vi "Basic Sweep.vi"(8 "error in (no error)":errorcluster, 11 "Wavepond in":refnum<class "Wavepond.lvclass">) -> (0 "error out":errorcluster, 3 "Wavepond out":refnum<class "Wavepond.lvclass">)   [LabVIEW 2015, in "Wavepond.lvclass"]
uses:
  Wavepond.lvclass
  Wavepond Commands.ctl
  Wavepond.lvclass/Wavepond.ctl
panel:
  out "standard output":string
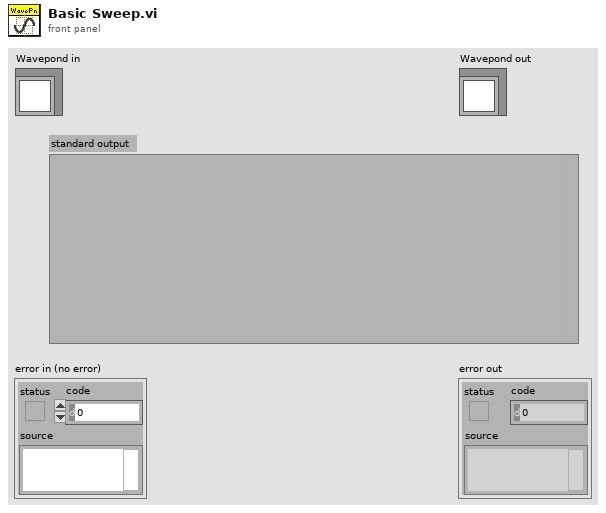
[diagram p1: front panel]
types:
  T1 = typedef "Wavepond.lvclass/Wavepond Commands.ctl" = enum16{"Initialize", "SetFrequency", "SetAtten", "WriteData", "EnableSweep", "SetLoopCnt", "SetClkDiv", "SelExtTrig", "SoftTrig", "En_SqWave"}
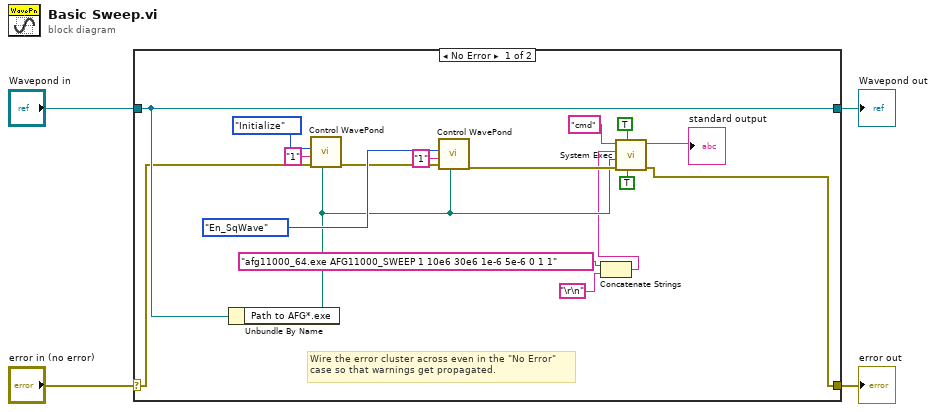
[diagram p0: block diagram]
diagram:
  n1 = case shown="No Error" "error in (no error)" {
    selector: "error in (no error)" -> [w19 w23]
    tunnel: [w10 w23] -> w3
    tunnel: [w21 w22] -> w1
    tunnel: "Wavepond in" -> [w21 w22]
    frame No Error {
      # "Wire the error cluster across even in the \"No Error\"\ncase so that warnings get propagated."
      n2 = Unbundle By Name(w21) -> ("Path to AFG*.exe"=w11:path)
      n3 = call "Control WavePond.vi"("working directory"=w11, "Error In"=w19, "Parameter"="1", "Command"=Wavepond_Commands."Initialize") -> ("Error Out"=w12:errorcluster)  [unwired: 5 in, 2 out]
      n4 = call "Control WavePond.vi"("working directory"=w11, "Error In"=w12, "Parameter"="1", "Command"=Wavepond_Commands."En_SqWave") -> ("Error Out"=w16:errorcluster)  [unwired: 5 in, 2 out]
      n5 = Concatenate Strings("afg11000_64.exe AFG11000_SWEEP 1 10e6 30e6 1e-6 5e-6 0 1 1" ("command line"), "\r\n") -> (w5:string)
      n6 = call <vilib>:"System Exec.vi"("run minimized? (F)"=TRUE, "wait until completion? (T)"=TRUE, "error in (no error)"=w16, "working directory"=w11, "standard input"=w5, "command line"="cmd") -> ("error out"=w10:errorcluster, "standard output"=→"standard output":string)  [unwired: 2 in, 2 out]
    }
    frame Error {
    }
  }
  "error out" <- w3
  "Wavepond out" <- w1
